vi "UHR-Fleezers Control (host) -TL - oscillation.vi"(0 "Tab Control":T5(tab)) -> ()   [LabVIEW 2013] (continued)
  in  "BD 2 Frequency 1 (MHz)":dbl=26.0 min=50.0 max=100.0 step=1.0 format="%#_6p"
  in  "Not-Interlacing Set":enum32{"Set 1", "Set 2", "Set 3"}(radio)
  in  "Interlace":bool=TRUE
  in  "Trap 2 ON":bool=TRUE
  in  "Trap 3 ON":bool
  in  "Scan axis (osc)":bool=TRUE
  in  "Osc. freq. (Hz)":dbl=32.0
  in  "Osc. amp. (MHz)":dbl=0.5 format="%1_3g"
  out "Coords":T8
  in  "Manipulation Scaling":cluster{"Horizontal":dbl, "Vertical":dbl}={"Horizontal"=0.075, "Vertical"=0.01}
  in  "Freq or Amp switch first":bool=TRUE
  in  "Swap F1 and F2":bool
  in  "Freq switch delay":u16
  in  "Amp switch delay":u16=5
  in  "Time Step (ms)":i64=1
  in  "MCL Step Increment (V_int)":dbl=3.0
  out "Time to Finish All (min)":dbl=0.122877 format="%#_2p"
  in  "Scan Speed (nm/s)":dbl=100.0
  in  "Scan Range (nm)":dbl=369.00000000000034
  in  "Step Size (nm)":dbl=1.0
  in  "MCL/AOM Scale Tweak":dbl=1.0
  in  "MCL Step Position Ratio":dbl=0.5
  in  "Move MCL Also?":bool=TRUE
  out "Final sep (nm)":dbl=4587.0
  out "Initial sep (nm)":dbl=4218.0
  out "Save index":dbl=22.0
  out "Final delta (MHz)":dbl=44.0
  out "Initial delta (MHz)":dbl=41.0
  out "Final freq. (MHz)":dbl=50.0
  out "Initial freq. (MHz)":dbl=53.0
  in  "Saved AOD Raster Scan Parameter Sets":T9(array[cluster])=[{"Scan Range AOD (nm) 2"=500.0, "Step Size AOD (nm) 2"=1.0, "Scan Speed AOD (nm/s) 2"=100.0, "Number of scans (AOD) 2"=1, "Label"="offset curve"}, {"Scan Range AOD (nm) 2"=420.0, "Step Size AOD (nm) 2"=1.0, "Scan Speed AOD (nm/s) 2"=100.0, "Number of scans (AOD) 2"=1, "Label"="hp raster check"}, {"Scan Range AOD (nm) 2"=6.8, "Step Size AOD (nm) 2"=0.34, "Scan Speed AOD (nm/s) 2"=0.34, "Number of scans (AOD) 2"=1, "Label"="3.4 kbp - 1 bp steps"}]
  in  "Load parameters":bool
  out "Scan Range (MHz)":dbl=-3.0000000000000027
  in  "Restart DMA? (AOD)":bool=TRUE caption="Restart DMA?"
  out "Incr. int (AOD)":i64=-7759651845
  out "Time/Scan (s) (AOD)":dbl=3.68631 format="%#_2p"
  out "Data points/scans":dbl=491508.0
  out "Data points/scan (f/b)":dbl=491508.0
  in  "Save scans":bool=TRUE
  out "AOD Scan I":u64 caption="Scan I"
  in  "Continuous AOD Scanning":bool caption="Continuous Scanning"
  in  "Abort AOD Scan":bool caption="Abort Scan"
  in  "Scan BD":bool=TRUE
  out "Cycles/step (AOD)":u64=666 format="%.3p"
  in  "Number of F/B Scans (AOD)":u16=1 min=1
  out "Scan steps (AOD)":u64=369
  out "Scan Increment (MHz)":dbl=-0.008152173913043485
  out "AOD Scanning":bool caption="Scanning"
  in  "Start AOD Scan":bool caption="Start Scan"
  out "N sets should be saved":dbl=24.5754
  out "Progress 2":u16(slide) caption="Progress" scale=0.0..100.0
  in  "Abort save 2":bool caption="Abort save"
  in  "Trap 1 Bead Size (nm)":dbl=2100.0
  in  "Trap 2 Bead Size (nm)":dbl=2100.0
  out "MCL Count":dbl=230502201.82069838
  in  "All FB On/Off":bool
  in  "AI2 to Setpoint":cluster{"Set 1":bool, "Set 2":bool}
  out "AI2 (V)":cluster{"Set 1":dbl, "Set 2":dbl}={"Set 1"=-0.0012207403790398877, "Set 2"=0.004577776421399579}
  in  "Reset Feedback":cluster{"Set 1":bool, "Set 2":bool}
  in  "PID Gains":T10={"Set 1"={"proportional gain (Kc)"=0, "integral gain (Kc*Ts/Ti)"=5, "derivative gain (Kc*Td/Ts)"=0}, "Set 2"={"proportional gain (Kc)"=0, "integral gain (Kc*Ts/Ti)"=5, "derivative gain (Kc*Td/Ts)"=0}}
  in  "Feedback On/Off":cluster{"Set 1":bool, "Set 2":bool}={"Set 1"=TRUE, "Set 2"=TRUE}
  in  "Reset Trap Pos. FB":bool
  in  "Tab Control 8":enum32{"Main Setting", "Details"}(tab)
  in  "Trap Pos FB Int Count":u16=100
  in  "Trap Pos. FB Gains":T11={"proportional gain (Kc)"=10.0, "integral gain (Kc*Ts/Ti)"=10.0, "derivative gain (Kc*Td/Ts)"=0.0} {"proportional gain (Kc)" format="%.11g"; "integral gain (Kc*Ts/Ti)" format="%.11g"; "derivative gain (Kc*Td/Ts)" format="%.11g"}
  in  "Trap Pos. FB Offset Factor":i64
  in  "Trap Pos FB Negate Action":bool
  in  "Trap Pos. FB Mult Factor":i64=33554432
  in  "Trap Pos. AI1 X Pre-scale":u16
  in  "Trap Pos. FB Range":T12={"output high"=0.999969482421875, "output low"=-1.0}
  out "Trap Pos FB Int Signal":fxp<+/-,24,9> format="%.18g"
  out "Trap Pos FB Int-Norm Signal":fxp<+/-,16,1> format="%.16g"
  in  "Set SP Using...":bool
  in  "Trap Pos FB Monitor\nT1 or T2":bool
  out "Trap X AI1 (DMA)":T13={"Set 1"=0.999969482421875, "Set 2"=0.999969482421875}
  in  "N El. to Ave.":dbl=10000.0
  out "Trap Pos FB Action":i64
  out "Mean T1 Position (nm)":dbl=-1.7479351299698465e-12 caption="Mean T1 (nm)" format="%0.2f"
  out "Trap 1 Position RMS (A)":dbl caption="RMS (Ang)"
  in  "Tab Control 3":enum32{"Timing", "MCL Scan", "Analog Out"}(tab)
  out "APD 2 Gate Late Counter":u32
  out "APD 2 Gate Relative Phase":i16
  in  "Phase Adj. (APD 2 Gate)":i16=20
  in  "Initial Phase Adjustment (APD 2 Gate)":i16=55
  out "APD 1 Gate Late Counter":u32
  in  "- phase (APD 1 Gate)":bool
  in  "+ phase (APD 1 Gate)":bool
  out "APD 1 Gate Relative Phase":i16
  in  "Phase Adj. (APD 1 Gate)":i16=20
  in  "Initial Phase Adjustment (APD 1 Gate)":i16=60
  in  "Save APD Data\nwith Trap Data":bool=TRUE
  out "APD FIFO Elements Remaining":u32
  in  "- phase (APD Acq)":bool
  in  "+ phase (APD Acq)":bool
  out "APD Acq Late Counter":u32
  out "APD Acq Relative Phase":i16
  in  "Phase Adj. (APD Acq)":i16=20
  in  "Initial Phase Adjustment (APD Acq)":i16
  in  "Invert APD Gate":bool caption="Invert Gate"
  in  "APD Gate OFF Count":u32=450 caption="Gate OFF Count"
  in  "APD Gate ON Count":u32=150 caption="Gate ON Count"
  in  "APD Gate":enum32{"ON", "OFF", "Interlace"}(radio)=enum."Interlace"
  in  "APD Integration Time (s)":dbl=0.01 caption="Integration Time (s)"
  out "APD Acq Rate (Hz)":dbl=100.0 caption="Rate (Hz)"
  out "APD Samples/FIFO Acq.":dbl=30.0
  out "APD Elements/DMA read":u32=60
  out "APD Int. Count":u32=400000 format="%.0p"
  in  "+ phase (APD 2 Gate)":bool
  in  "- phase (APD 2 Gate)":bool
  in  "Tab Control 5":enum32{"PSD X", "PSD Y", "Other Data Channel"}(tab)
  out "Data map":dbl[][](graph)
  in  "Channel":i32=4
  in  "Abort MCL Scan":bool
  out "MCL Scan I":u64
  out "MCL Scanning":bool
  in  "Start MCL Scan":bool
  out "wait to reset values":bool
  in  "Tab Control 4":enum32{"Scan Settings", "MCL FPGA Loop Timing"}(tab)
  out "Total Time (s)":dbl=48.0
  in  "Scan lines (y)":u64=20
  in  "Fast Scan Dir":bool=TRUE
  in  "2D or 1D Scan":bool=TRUE
  out "Initial X":dbl
  out "Initial Y":dbl
  out "Time/f+b scan (s) (MCL)":dbl=2.4 caption="Time/scan (s)"
  in  "Number of scans (MCL)":u64=1 caption="Scans"
  in  "Scan steps (MCL)":u64=40 caption="Scan steps (x)"
  in  "N APD Samp/step":dbl=3.0
  in  "Scan Range (V)\n(of steps)":dbl=3.5
  in  "Restart DMA? (MCL)":bool=TRUE caption="Restart DMA?"
  in  "Continuous MCL Scanning":bool caption="Cont. Scanning"
  in  "Center Scan":bool=TRUE
  in  "Save Data (MCL)":bool=TRUE caption="Save Data"
  out "Actual Incr. int (MCL)":i16=294 caption="Incr. int"
  out "Desired incr (int)":dbl=294.0628205128205
  out "Desired Scan Incr (V)":dbl=0.08974358974358974
  out "N sets should be saved (MCL)":dbl=160.0 caption="N sets should be saved"
  out "Data points/scans (MCL)":dbl=4800.0 caption="Data points/scans"
  out "Data points/scan (f+b)":dbl=240.0 caption="points/scan (f+b)"
  out "Cycles/step (MCL)":u64=2000 caption="Cycles/step" format="%.0p"
  out "Actual MCL Inc (V)":dbl=0.08972441785943175
  in  "Phase adjust (MCL)":i16 caption="Phase adjust"
  out "Relative Phase (MCL)":i16 caption="Relative Phase"
  in  "Initial Phase Adj. (MCL)":i16 caption="Initial Phase Adj."
  in  "Update Count (MCL)":u32=600
  in  "+ phase (MCL)":bool
  in  "- phase (MCL)":bool
  out "MCL Late Counter":u32
  in  "APD 1 AO Mult.":i16=1 min=1
  in  "APD 2 AO Mult.":i16=1 min=1
  in  "Tab Control 7":enum32{"Green FB Signals", "Slow MCL Scan"}(tab)
  out "Green FB Plot":dbl(graph)=10.0
  out "MCL Scan 2":cluster{"Begin (V)":dbl, dbl, dbl[]}(graph)
  out "MCL Scan":cluster{"Begin (V)":dbl, dbl, dbl[]}(graph)
  in  "Green laser mode":enum32{"Laser ON", "Laser OFF", "Interlace"}(radio)
  in  "GI Frequency, ON count":u32=150 min=1 step=1
  in  "Invert GI":bool
  out "GI Late Counter":u32
  in  "Phase adj. (GI)":i16=5
  out "GI relative phase":i16
  in  "+ phase (GI)":bool
  in  "Initial Phase Adjustment (GI)":i16=19
  in  "GI Frequency, OFF count":u32=450 min=1 step=1
  in  "- phase (GI)":bool
  out "Green FB Signals (V)":cluster{"Y":dbl, "X":dbl, "Sum":dbl}={"Y"=1.0, "X"=1.0, "Sum"=10.0}
  out "Relative phase (Green FB)":i16
  in  "+ phase (Green FB)":bool
  in  "- phase (Green FB)":bool
  in  "Green FB Count":u32=600
  in  "Phase adj. (Green FB)":i16=10
  in  "Initial Phase Adjustment (Green FB)":i16=50
  in  "Green FB On/Off":bool
  in  "Current When FB OFF (%)":dbl=10.0 min=0.0 max=100.0 step=1.0
  in  "Green int current ON count adj":u32=150
  in  "Green FB Gains":T14={"proportional gain (Kc)"=10, "integral gain (Kc*Ts/Ti)"=5, "derivative gain (Kc*Td/Ts)"=0}
  in  "Green FB Setpoint (mV)":dbl=100.0
  in  "- phase (GI) 2":bool
  in  "Initial Phase Adjustment (GI) 2":i16=-100
  in  "+ phase (GI) 2":bool
  out "GI relative phase 2":i16
  in  "Phase adj. (GI) 2":i16=20
  out "GI Late Counter 2":u32
  in  "Trap Position FIFO Depth":u32=300000 format="%.0p"
  in  "# Samples/trap":u32=20000 format="%.0p"
  out "Trap AI Elements/DMA read":u32=320000 format="%.0p"
  out "Ave. Rate (Hz)":dbl=200000.0 format="%#_6p"
  out "Trap AI FIFO El. Rem.":u32 format="%.0p"
  in  "Phase adj. (AI1)":i16
  out "Relative phase (AI1)":i16
  in  "+ phase (AI1)":bool
  in  "- phase (AI1)":bool
  out "Late Counter (AI1)":u32
  in  "Initial Phase Adjustment (AI1)":i16=180
  out "AI rate (Hz)":dbl=200000.0 format="%#_6p"
  in  "AI Count (ticks)":u32=200
  out "# Samples/channel":u32=40000 format="%.0p"
  in  "Trap AI FIFO Depth":u32=340000 format="%.0p"
  in  "Detector Type":string(combo)="UCB Fleezers 052511"
  in  "N Acq Sets (Traps + Fl.)":i16=3
  in  "Sets to FIFO (Traps)":T15={"Set 1"=TRUE, "Set 2"=TRUE, "Set 3"=FALSE}
  in  "FPGA Ave.":dbl=1.0 min=1.0 step=1.0
  out "Ave. Period (s)":dbl=5e-06 format="%#_6p"
  out "DMA Update Period (s)":dbl=0.3
  out "FPGA Averaging":bool
  out "Trap Sets":u32=2
  out "Counts/DMA":dbl=12000000.0 format="%#_6p"
  out "Trap Pos FIFO El Remaining":u32=141
  out "Trap Pos Elements/DMA read":u32=120000 format="%.0p"
  out "Trap AI FIFO Timeout":u16
  out "Trap Pos FIFO Timeout":u16
  out "Waveform Chart":i32(graph)=320000
  out "error out 2":errorcluster
  in  "Lost Tether Alarm Threshold (pN)":dbl=0.5
  in  "AOM X Cal (nm/MHz)":dbl=168.33
  in  "MCL X Cal (nm/V)":dbl=1070.0
  out "X RF Amplitude Limits (%)":T16={"Minimum"=0.0, "Maximum"=50.0, "Increment"=1.0}
  out "X RF Frequency Limits (MHz)":T16={"Minimum"=50.0, "Maximum"=100.0, "Increment"=1.0}
  out "Y RF Frequency Limits (MHz)":T16={"Minimum"=50.0, "Maximum"=100.0, "Increment"=1.0}
  out "Y RF Amplitude Limits (%)":T16={"Minimum"=0.0, "Maximum"=50.0, "Increment"=1.0}
  in  "Manip. X?":bool=TRUE
  in  "Manip. Y?":bool
  in  "Force Manip Abort":bool
  out "Read cal error":errorcluster
  in  "DAQ Delay (ms)":u32=1000
  in  "Start Scan":bool
  in  "Scan axis":bool
  in  "Osc. amp. (V)":dbl=5.0
  in  "Osc. center (V)":dbl=5.0
  in  "Osc. freq. (Hz) 2":dbl=1.0
  in  "MCL Mode":u16(ring) items=["Manual Positioning", "Sinusoidal Wave", "Linear Scan"]
  in  "Begin (V)":dbl
  in  "End (V)":dbl=10.0
  in  "N Points":dbl=20.0
  in  "Delay to Interlace (s)":dbl
  in  "Delayed Interlace Start":bool
  in  "Read Lateness and Rel Phase":bool
  out "Vec Mean of T1 T2":dbl[](array[numeric])=[nan, nan]
  in  "Cal read wait (s)":u32=5
  out "Time tether formed":timestamp=timestamp(3371146929.513132 s since 1904-01-01)
  in  "Chemyx Syringe Pump Serial Port":refnum<visa-resource-name>="ASRL3::INSTR"
  in  "Limit Min (MHz)":dbl=10.0 caption="Min (MHz)"
  in  "Limit Max (MHz)":dbl=16.0 caption="Max (MHz)"
  in  "Limits Enable":bool=TRUE caption="Enable"
  out "AI labels":string[](array[string])=["T1 Y", "T1 X", "T1 Sum", "T2 Y", "T2 X", "T2 Sum", "T1 FB X", "T2 FB Sum", "T2 FB X", "T2 FB Sum", "PSD Y", "PSD X", "PSD Sum"]
  in  "Save Trap Pos. Data":bool=TRUE
  in  "ESP Port":refnum<visa-resource-name>="COM4"
  in  "Axis 3":string="0.00500\r\n"
  in  "Axis 2":string="0.00500\r\n"
  in  "Axis 1":string="0.00500\r\n"
  in  "Axis 3":string="0.20000\r\n"
  in  "Axis 2":string="0.20000\r\n"
  in  "Axis 1":string="0.20000\r\n"
  in  "Activate Joystick":bool
  in  "ESP ZL-Limit":string="-0.09900"
  in  "ESP ZR-Limit":string="0.09900"
  in  "error in":errorcluster
  out "error out":errorcluster
  # "Save Positions of Cambers"
  # "After"
  # "During"
  # "Trap On?"
  # "BD Flow ON?"
  # "Samp Flow ON?"
  # "1"
  # "2"
  # "Trap Display:"
  # "APD Display:"
  # "originally 10k"
  # "Data Saving"
  # "Trap Manipulation"
  # "DAQ"
  # "Central frequency 80 MHz"
  # "F9"
  # "F10"
  # "Bead Calibration"
  # "Current Location"
  # "Select the chamber to go to"
  # "F4"
  # "Press F12 to move stage\nwith the mouse. F12 to cancel."
  # "F5"
  # "F6"
  # "F7"
  # "F8"
  # "Harvard Pump\n(sample channel for flow exp)"
  # "Chemyx Pump 2"
  # "Units: \n1 = ml/m\n2 = ml/h\n3 = ul/m\n4 = ul/h"
  # "Rate param is ul/h\nVolume param is ul"
  # "X"
  # "Y"
  # "Oscillate Set freq. (debugging)"
  # "BD 1"
  # "BD 2"
  # "AOD Raster Scan"
  # "Approx. trap separations"
  # "X"
  # "Y"
  # "DON'T TURN ON\nUNTIL YOU CLOSE\nTHE LOOP"
  # "FPGA\nreading"
  # "DMA\ntransfer"
  # "APD Gates"
  # "APD 2"
  # "APD 1"
  # "X"
  # "2D"
  # "Y"
  # "1D"
  # "Green FB Measurement"
  # "Green Laser Interlacing"
  # "Digital Gate"
  # "Current Analog Control"
  # "was 87"
  # "originally 600k"
  # "Total AI Rates (NOT rates/trap)"
  # "originally 20k"
  # "(Samples/trap x Trap Sets)"
  # "(Samples/channel x\n8 if averaging (8 channels)\n4 if no averaging)"
  # "Trap 1"
  # "Trap 2"
  # "Flour./Trap 3"
  # "External Video Window"
  # "MCL Position Debugging"
  # "Temporary Control Storage\n(these used to be somewhere else, still want to keep them)"
  # "Y"
  # "X"
  # "Trap Position Difference Limits"
  # "Joystick Control"
  # "Setting Limit for the z-axis"
  # "Errors detected in determing Current Location"
  # "High Jog Velocity"
  # "Low Jog Velocity"
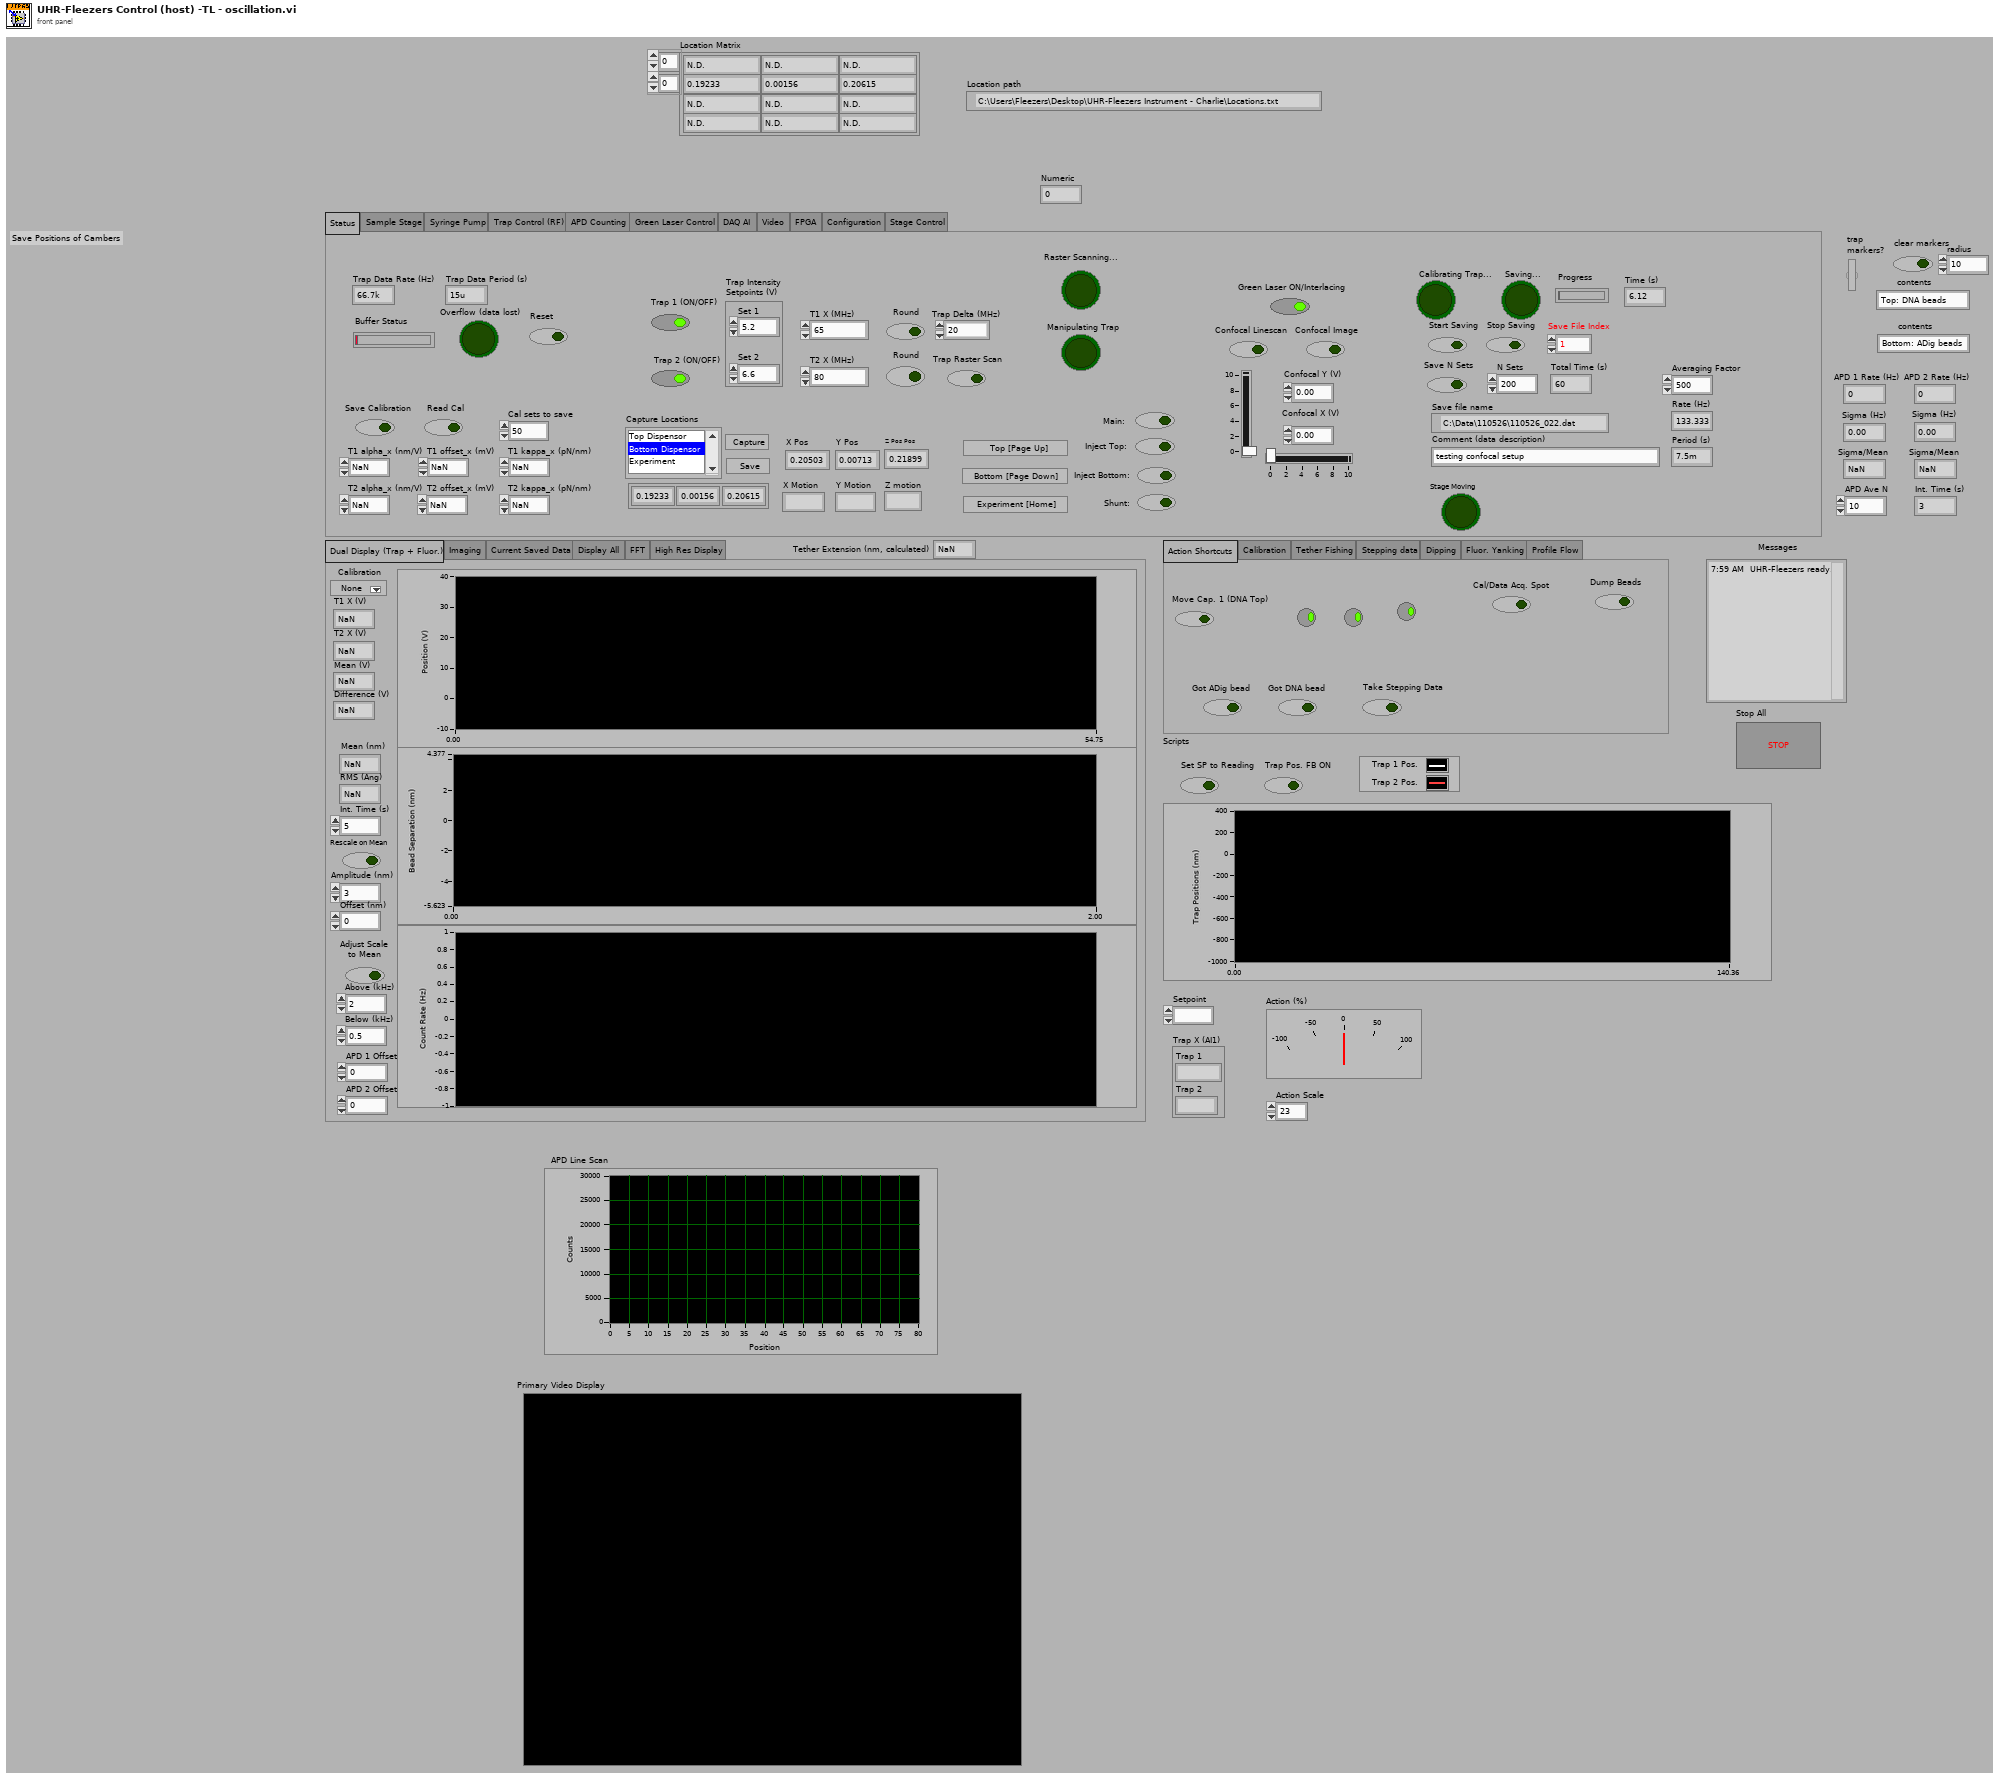
[diagram p1: front panel]
types:
  T1 = cluster{"Trap 1":fxp<+/-,16,1>, "Trap 2":fxp<+/-,16,1>}
  T2 = enum32{"Action Shortcuts", "Calibration", "Tether Fishing", "Stepping data", "Dipping", "Fluor. Yanking", "Profile Flow"}
  T3 = typedef "IMAQ Image.ctl" = refnum<image>
  T4 = enum32{"Dual Display (Trap + Fluor.)", "Imaging", "Current Saved Data", "Display All", "FFT", "High Res Display"}
  T5 = enum32{"Status", "Sample Stage", "Syringe Pump", "Trap Control (RF)", "APD Counting", "Green Laser Control", "DAQ AI", "Video", "FPGA", "Configuration", "Stage Control"}
  T6 = cluster{"Pump 1":cluster{"Diameter (mm)":dbl, "Units":dbl, "Volume":dbl, "Rate":dbl}, "Pump 2":cluster{"Diameter (mm)":dbl, "Units":dbl, "Volume":dbl, "Rate":dbl}, "Pump 3":cluster{"Diameter (mm)":dbl, "Units":dbl, "Volume":dbl, "Rate":dbl}}
  T7 = enum32{"IR Laser Interlacing (Direct RF Board Control Method)", "AOD Raster Scan", "Feedback on Trap Intensity", "Feedback on Trap Position"}
  T8 = typedef "LVPoint32TypeDef.ctl" = cluster{"Horizontal":i32, "Vertical":i32}
  T9 = cluster{"Scan Range AOD (nm) 2":dbl, "Step Size AOD (nm) 2":dbl, "Scan Speed AOD (nm/s) 2":dbl, "Number of scans (AOD) 2":u16, "Label":string}[]
  T10 = cluster{"Set 1":cluster{"proportional gain (Kc)":i16, "integral gain (Kc*Ts/Ti)":i16, "derivative gain (Kc*Td/Ts)":i16}, "Set 2":cluster{"proportional gain (Kc)":i16, "integral gain (Kc*Ts/Ti)":i16, "derivative gain (Kc*Td/Ts)":i16}}
  T11 = cluster{"proportional gain (Kc)":fxp<+/-,16,8>, "integral gain (Kc*Ts/Ti)":fxp<+/-,16,8>, "derivative gain (Kc*Td/Ts)":fxp<+/-,16,8>}
  T12 = cluster{"output high":fxp<+/-,16,1>, "output low":fxp<+/-,16,1>}
  T13 = cluster{"Set 1":fxp<+/-,16,1>, "Set 2":fxp<+/-,16,1>}
  T14 = cluster{"proportional gain (Kc)":i16, "integral gain (Kc*Ts/Ti)":i16, "derivative gain (Kc*Td/Ts)":i16}
  T15 = cluster{"Set 1":bool, "Set 2":bool, "Set 3":bool}
  T16 = typedef "LVMinMaxIncTypeDef.ctl" = cluster{"Minimum":dbl, "Maximum":dbl, "Increment":dbl}
  T17 = typedef "Image Type" = u32
  T18 = typedef "nirio_resource_hc.ctl" = tag
  T19 = typedef "openfpgaref.8.6.ctl" = refnum<k20>
  T20 = enum16{"CONNECT", "INITIALIZE VALVES", "DISCONNECT", "MOVE VALVE"}
  T21 = cluster{"New Image":T3, "New Image":T3, "New Image":T3, "New Image":T3}
  T22 = cluster{"Location Matrix[0]":string, "Location Matrix[1]":string, "Location Matrix[2]":string}
  T23 = enum16{"open", "replace", "create", "open or create", "replace or create", "replace or create with confirmation"}
  T24 = typedef "XDNodeRunTimeDep.lvlib/timing_clust.ctl" = cluster{"Expected End [f-1]":u64, "Actual End [f-1]":u64, "Finished Late? [f-1]":bool, "Expected End [i-1]":u64, "Actual End [i-1]":u64, "Finished Late? [i-1]":bool, "Expected Start [i]":u64, "Actual Start [i]":u64, "Expected Start [f]":u64, "Actual Start [f]":u64, "Source Name":string, "Structure Name":string, "Period":i64, "Deadline":i64, "Offset":i64, "Start":i64, "Priority":i32, "Timeout":i32, "Mode":T25, "Wakeup Reason":T26, "Error":errorcluster, "Source Type":string, "Secondary Source Type":string, "Global End Time":u64, "Global Start Time":u64, "Frame Duration":u64, "Iteration Duration":u64, "Assigned CPU":i32, "I/O Scan Engine Mode":u32}
  T25 = typedef "XDNodeRunTimeDep.lvlib/nitl_modes.ctl" = enum32{"No Change", "Process missed periods, maintain original phase", "Discard missed periods, maintain original phase", "Process missed periods, ignore original phase", "Discard missed periods, ignore original phase"}
  T26 = typedef "XDNodeRunTimeDep.lvlib/wakeup.ctl" = enum32{"Normal", "Aborted", "Asynchronous wakeup", "Timing source error", "Timed loop error", "Timeout"}
  T27 = cluster{"[0]":i32, "[1]":i32, "[2]":i32, "[3]":i32}
  T28 = cluster{"[0]":i32, "[1]":i32, "[2]":i32, "[3]":i32}[]
  T29 = enum16{"big-endian, network order", "native, host order", "little-endian"}
  T30 = cluster{"Scan Range AOD (nm) 2":dbl, "Step Size AOD (nm) 2":dbl, "Scan Speed AOD (nm/s) 2":dbl, "Number of scans (AOD) 2":u16, "Label":string}
  T31 = cluster{"[0]":dbl, "[1]":dbl, "[2]":dbl, "[3]":dbl, "[4]":dbl, "[5]":dbl}
  T32 = cluster{"Diameter (mm)":dbl, "Units":dbl, "Volume":dbl, "Rate":dbl}
  T33 = cluster{"Left":i32, "Top":i32, "Width":u32, "Height":u32}
  T34 = cluster{cluster{"Left":i32, "Top":i32, "Width":u32, "Height":u32}}[]
  T35 = enum32{"Normal Display", "Dual Display (APD)", "FFT", "High Res Display"}
  T36 = cluster{"Origin Pixel":cluster{"X":sgl, "Y":sgl}, "Angle Relative to Horizontal (deg)":sgl, "Axis Reference":u32}
  T37 = typedef "Simple Grid Descriptor" = cluster{"X Step":sgl, "Y Step":sgl, "Unit":T38}
  T38 = typedef "Image Unit" = enum32{"Undefined", "Angström", "Micrometer", "Millimeter", "Centimeter", "Meter", "Kilometer", "Microinch", "Inch", "Feet", "Nautical miles", "Standard miles", "Steps"}
  T39 = cluster{"averaging mode":u16, "weighting mode":u16, "number of averages":u32}
  T40 = cluster{"dB On (F)":bool, "unwrap phase (F)":bool, "convert to degree (F)":bool}
  T41 = cluster{string, string, string, string, string, string, string, string}
  T42 = cluster{string, string, string, string, string, string, string, string, string, string, string, string}
  T43 = cluster{string, string, string, string, string, string, string, string, string, string, string, string, string}
  T44 = cluster{string, string, string, string, string, string, string, string, string, string, string, string, string, string}
  T45 = cluster{"BD 1 Frequency 1 (MHz)":dbl, "BD 1 Frequency 2 (MHz)":dbl}
  T46 = cluster{"f0":dbl, "df":dbl, "magnitude":dbl[]}[][]
  T47 = cluster{"Green FB Ch 0":i16, "Green FB Ch 1":i16, "Green FB Ch 2":i16}
  T48 = cluster{"Green FB Ch 0":dbl, "Green FB Ch 1":dbl, "Green FB Ch 2":dbl}
diagram:
  w67 = T17 2 items=["Grayscale (U8)", "Grayscale (I16)", "Grayscale (SGL)", "Complex (CSG)", "RGB (U32)", "HSL (U32)", "RGB (U64)", "Grayscale (U16)"] ("Image Type")
  w124 = cluster{"output high":i16, "output low":i16} {"output high"=3000, "output low"=0} ("FB output range 1")
  w198 = 10.0 ("y")
  w197 = 32767.0 ("y")
  w213 = 6.0  # clock mult.
  w214 = 49152000.0  # TCXO frequ.
  # "Initialize location matrix"
  n1 = Build Array("DIO count 1 (ticks)", "DIO count 2 (ticks)", "DIO count 3 (ticks)") -> (w113:u32[])
  n2 = Multiply(x="APD Integration Time (s)", y=40000000.0) -> (x*y=w131:dbl)
  n3 = Reciprocal(x="APD Integration Time (s)") -> (1/x=w128:dbl)
  n4 = local write "APD Acq Rate (Hz)"(w128) -> ()
  n5 = local read "AO1"() -> (w192:dbl)
  n6 = local read "AO2"() -> (w191:dbl)
  n7 = To Unsigned Long Integer(number=w131) -> (unsigned 32bit integer=w130:u32)
  "APD Int. Count" <- w130
  n8 = local read "Scan Increment (MHz)"() -> (w209:dbl)
  n9 = local read "Continuous MCL Scanning"() -> (w179:bool)
  n10 = local read "Fast Scan Dir"() -> (w178:bool)
  n11 = local read "Trap Intensity\nSetpoints (V)"() -> (w228:cluster{"Set 1":dbl, "Set 2":dbl})
  n12 = local read "Number of scans (MCL)"() -> (w180:u64)
  n13 = Multiply(x=w192, y=w197) -> (x*y=w194:dbl)
  n14 = Multiply(x=w191, y=w197) -> (x*y=w196:dbl)
  n15 = Divide(x=w194, y=w198) -> (x/y=w193:dbl)
  n16 = Divide(x=w196, y=w198) -> (x/y=w195:dbl)
  n17 = To Word Integer(number=w193) -> (16bit integer=w190:i16)
  n18 = To Word Integer(number=w195) -> (16bit integer=w189:i16)
  n19 = Not(x=w178) -> (.not. x?=w173:bool)
  n20 = local read "Cycles/step (MCL)"() -> (w181:u64)
  n21 = Multiply(x=w209, y=1000.0) -> (x*y=w216:dbl)
  n22 = local read "Scan steps (MCL)"() -> (w182:u64)
  n23 = local write "Trap Pos FIFO Timeout"(u16 0 ("Trap Pos FIFO Timeout")) -> ()
  n24 = local read "Desired Scan Incr (V)"() -> (w184:dbl)
  n25 = Scale By Power Of 2(n=48, x=w216) -> (x*2^n=w217:dbl)
  n26 = Multiply(x=w214, y=w213) -> (x*y=w212:dbl)
  n27 = Divide(x=w217, y=w212) -> (x/y=w211:dbl)
  n28 = local read "Number Interlace Sets"() -> (w106:u8)
  n29 = Split 1D Array(array=w113, index=w106) -> (first subarray=w115:u32[])  [unwired: 1 out]
  n30 = Add Array Elements(numeric array=w115) -> (sum=w114:u32)
  n31 = property on="AI Count (ticks)" class="DigNum (strict)"("Val(Sgnl)"="AI Count (ticks)") -> ()  [unwired: 2 in, 2 out]
  n32 = local read "# Samples/channel"() -> (w201:u32)
  n33 = local read "Number of F/B Scans (AOD)"() -> (w202:u16)
  n34 = To Quad Integer(1:w211) -> (0:w208:i64)
  n35 = local read "Not-Interlacing Set"() -> (w105:enum32{"Set 1", "Set 2", "Set 3"})
  n36 = To Unsigned Byte Integer(number=w105) -> (unsigned 8bit integer=w111:u8)
  n37 = Index Array(array=w113, index=w111) -> (element=w112:u32)
  n38 = local read "Feedback On/Off"() -> (w231:cluster{"Set 1":bool, "Set 2":bool})
  n39 = local read "PID Gains"() -> (w223:T10)
  n40 = Divide(x=40000000.0, y="AI Count (ticks)") -> (x/y=w170:dbl)
  n41 = Multiply(x=w184, y=32767.0) -> (x*y=w186:dbl)
  n42 = local read "Scan steps (AOD)"() -> (w207:u64)
  n43 = local read "All FB On/Off"() -> (w232:bool)
  n44 = local read "Cycles/step (AOD)"() -> (w206:u64)
  n45 = local write "AI rate (Hz)"(w170) -> ()
  n46 = Divide(x=w186, y=10.0) -> (x/y=w185:dbl)
  n47 = Multiply(x=w207, y=w206) -> (x*y=w205:u64)
  n48 = Multiply(x=3276.7, y=w228) -> (x*y=w227:cluster{"Set 1":dbl, "Set 2":dbl})
  n49 = To Word Integer(number=w185) -> (16bit integer=w183:i16)
  n50 = Multiply(x=w205, y=u64 2) -> (x*y=w203:u64)
  n51 = local read "Sets to FIFO (Traps)"() -> (w235:T15)
  n52 = Divide(x=w170, y="FPGA Ave.") -> (x/y=w171:dbl)
  n53 = To Word Integer(number=w227) -> (16bit integer=w226:cluster{"Set 1":i16, "Set 2":i16})
  n54 = xnode "Open FPGA VI Reference"("resource name"=T18 "RIO0") -> ("FPGA VI Reference Out"=w220:T19)  [unwired: 1 in, 1 out]
  n55 = Unbundle By Name(w223) -> ("Set 1"=w222:T14, "Set 2"=w221:T14)
  n56 = Multiply(x=w203, y=w202) -> (x*y=w200:u64)
  n57 = local write "Ave. Rate (Hz)"(w171) -> ()
  n58 = Divide(x=w200, y=w201) -> (x/y=w199:dbl)
  n59 = Unbundle By Name(w226) -> ("Set 1"=w225:i16, "Set 2"=w224:i16)
  n60 = local read "2D or 1D Scan"() -> (w125:bool)
  n61 = local write "Data points/scans"(w200) -> ()
  n62 = local read "Scan BD"() -> (w218:bool)
  n63 = And(x=w231, y=w232) -> (x .and. y?=w230:cluster{"Set 1":bool, "Set 2":bool})
  n64 = local write "Data points/scan (f/b)"(w203) -> ()
  n65 = Reciprocal(x=w171) -> (1/x=w172:dbl)
  n66 = local read "N Acq Sets (Traps + Fl.)"() -> (w164:i16)
  n67 = local write "N sets should be saved"(w199) -> ()
  n68 = Unbundle By Name(w230) -> ("Set 1"=w234:bool, "Set 2"=w233:bool)
  n69 = local read "Interlace"() -> (w107:bool)
  n70 = Select(t=w114, s=w107, f=w112) -> (s? t:f=w104:u32)
  n71 = local write "Update Count (MCL)"(w104) -> ()
  n72 = local write "Total Counts (ticks)"(w104) -> ()
  n73 = xnode "Invoke Method"("FPGA VI Reference In"=w220) -> ("FPGA VI Reference Out"=w123:T19, "error out"=w142:errorcluster)  [unwired: 1 in]
  n74 = local write "Ave. Period (s)"(w172) -> ()
  n75 = property on="2D or 1D Scan" class="Bool (strict)"("Val(Sgnl)"=w125) -> ()  [unwired: 2 in, 2 out]
